vi "insert action in sequence.vi"(7 "index":i32, 8 "error in (no error)":errorcluster, 9 "new action":refnum<class "action configuration.lvclass">, 10 "sequence name":string, 11 "Simple Sequencer TBM configuration in":refnum<class "Simple Sequencer TBM configuration.lvclass">) -> (0 "error out":errorcluster, 3 "Simple Sequencer TBM configuration out":refnum<class "Simple Sequencer TBM configuration.lvclass">)   [LabVIEW 2014, in "Simple Sequencer TBM configuration.lvclass"]
doc: "Inserts the given action into the specified sequence at the specified index."
uses:
  Simple Sequencer TBM configuration.lvclass
  sequencer parent classes/action configuration parent/action configuration.lvclass
  Simple Sequencer TBM configuration.lvclass/Simple Sequencer TBM configuration.ctl
  <vilib>/NI/Configuration Framework/serializable configuration/NISE_CEF_serializable configuration.lvclass
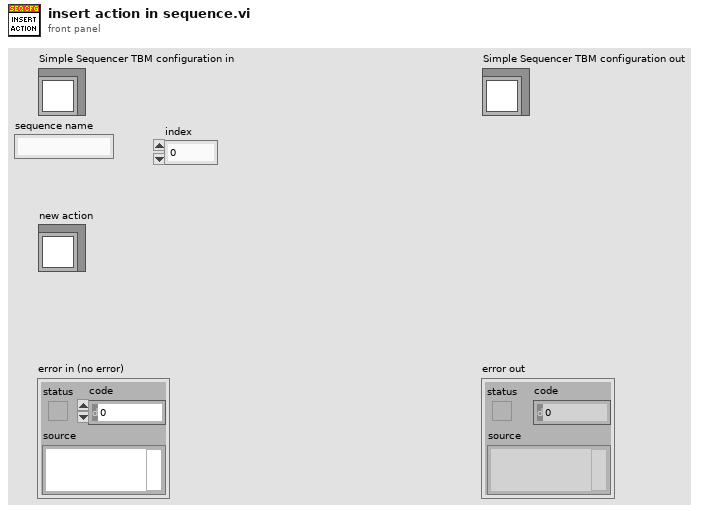
[diagram p1: front panel]
types:
  T1 = typedef "Simple Sequencer TBM configuration.lvclass/sequence definition.ctl" = cluster{"sequence name":string, "action configs":refnum<class "action configuration.lvclass">[]}
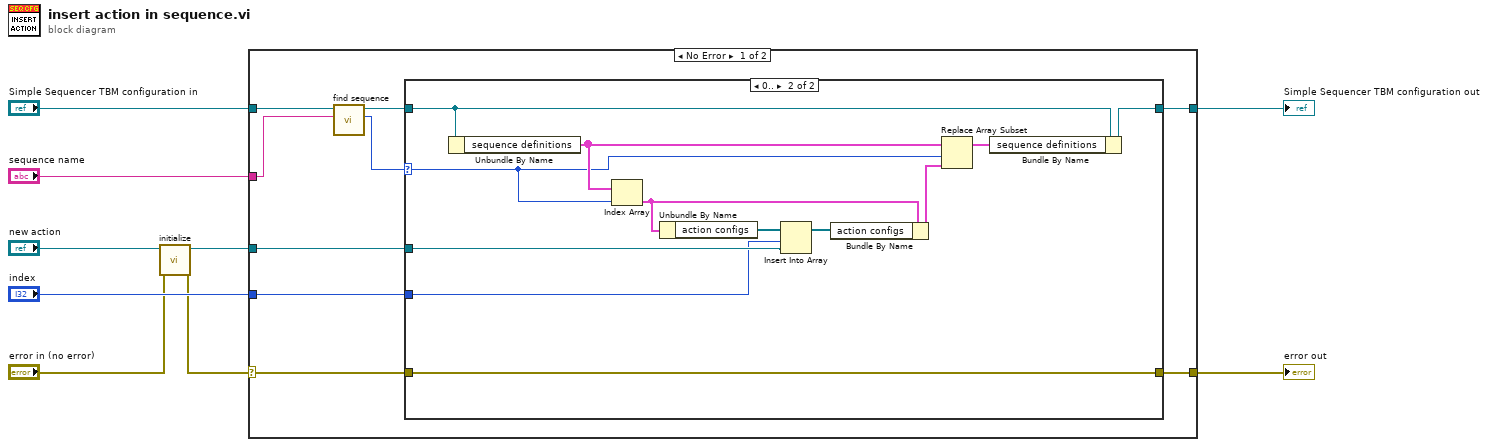
[diagram p0: block diagram]
diagram:
  n1 = call <vilib>:"initialize.vi"("error in"="error in (no error)", "configuration in"="new action") -> ("error out"=w1:errorcluster, "configuration out"=w3:refnum<class "action configuration.lvclass">)  [unwired: 7 in, 1 out]
  n2 = case shown="No Error" w1 {
    selector: w1 -> [w14 w34]
    tunnel: [w13 w34] -> w7
    tunnel: [w11 w33] -> w8
    tunnel: "Simple Sequencer TBM configuration in" -> [w18 w33]
    tunnel: "sequence name" -> [w17 _]
    tunnel: w3 -> [w12 _]
    tunnel: "index" -> [w10 _]
    frame No Error {
      n3 = call "find sequence.vi"("sequence name"=w17, "Simple Sequencer TBM configuration in"=w18) -> ("index"=w16:i32, "Simple Sequencer TBM configuration out"=w15:refnum<class "Simple Sequencer TBM configuration.lvclass">)  [unwired: 8 in]
      n4 = case shown="0.." w16 {
        selector: w16 -> [_ w29]
        tunnel: w15 -> [w19 w27]
        tunnel: w14 -> [w20 w32]
        tunnel: [w20 w32] -> w13
        tunnel: w12 -> [_ w22]
        tunnel: [w19 w25] -> w11
        tunnel: w10 -> [_ w21]
        frame ..-1 {
          # "#todo throw error not found"
        }
        frame 0.. {
          n5 = Unbundle By Name(w27) -> ("sequence definitions"=w30:T1[])
          n6 = Index Array(array=w30, index=w29) -> (element=w31:T1)
          n7 = Unbundle By Name(w31) -> ("action configs"=w24:refnum<class "action configuration.lvclass">[])
          n8 = Insert Into Array(array=w24, index=w21, new element=w22) -> (w23:refnum<class "action configuration.lvclass">[])
          n9 = Bundle By Name(cluster=w31, "action configs"=w23) -> (w28:T1)
          n10 = Replace Array Subset(array=w30, new element=w28, index=w29) -> (w26:T1[])
          n11 = Bundle By Name(cluster=w27, "sequence definitions"=w26) -> (w25:refnum<class "Simple Sequencer TBM configuration.lvclass">)
        }
      }
    }
    frame Error {
    }
  }
  "error out" <- w7
  "Simple Sequencer TBM configuration out" <- w8
